vi "LVClass_HasoSlopes Set Slopes X.vi"(0 "HasoSlopes in":refnum<class "HasoSlopes.lvclass">, 5 "Slopesx":sgl[][](array[numeric]), 11 "error in (no error)":errorcluster) -> (4 "HasoSlopes out":refnum<class "HasoSlopes.lvclass">, 15 "error out":errorcluster)   [LabVIEW 2020, in "HasoSlopes.lvclass"]
doc: "HasoSlopes X coordinates getter.\n\n--------------------------------------------------------------------------------\n\n<B>HasoSlopesIn </B> : HasoSlopes object.\n<B>HasoSlopesOut </B> : HasoSlopes object.\n<B>slopes_x </B> : 2D slopes X buffer.\n<B>ErrorIn </B> : Error\n<B>ErrorOut </B> : Error\n\n--------------------------------------------------------------------------------"
uses:
  HasoSlopes.lvclass
  HasoSlopes.lvclass/HasoSlopes.ctl
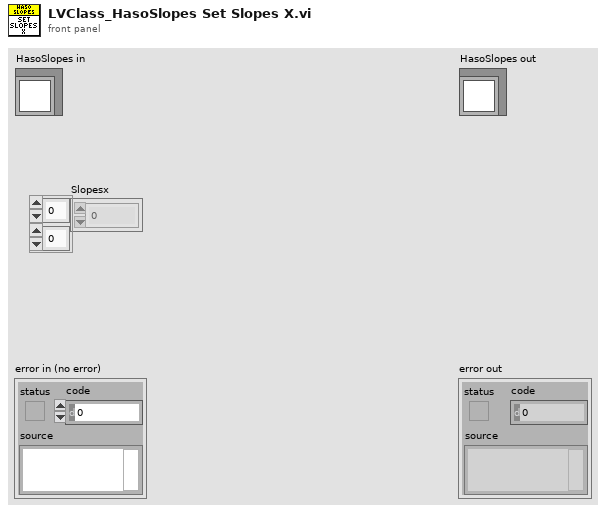
[diagram p1: front panel]
types:
  T1 = typedef "Point2D.ctl" = cluster{"X":u32, "Y":u32}
  T2 = typedef "Point2Df.ctl" = cluster{"X":sgl, "Y":sgl}
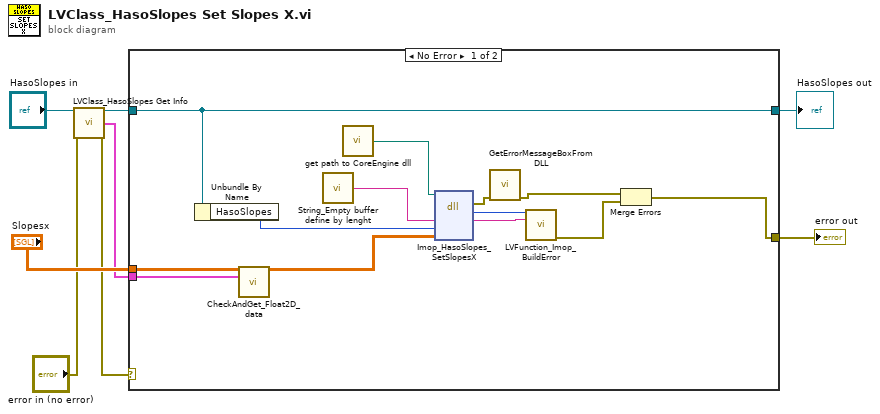
[diagram p0: block diagram]
diagram:
  n1 = call "LVClass_HasoSlopes Get Info.vi"("HasoSlopes in"="HasoSlopes in", "error in (no error)"="error in (no error)") -> ("HasoSlopes out"=w1:refnum<class "HasoSlopes.lvclass">, "dimension"=w5:cluster{"size":T1, "step":T2}, "error out"=w3:errorcluster)  [unwired: 9 in, 2 out]
  n2 = case shown="No Error" w3 {
    selector: w3 -> [_ w23]
    tunnel: [w12 w23] -> w8
    tunnel: [w15 w22] -> w7
    tunnel: w1 -> [w15 w22]
    tunnel: "Slopesx" -> [w11 _]
    tunnel: w5 -> [w9 _]
    frame No Error {
      n3 = Unbundle By Name(w15) -> ("HasoSlopes"=w18:i32)
      n4 = call "CheckAndGet_Float2D_data.vi"("data in"=w11, "Dimensions_um"=w9) -> ("data out"=w10:sgl[][])  [unwired: 13 in]
      n5 = call "String_Empty buffer define by lenght.vi"() -> ("Empty buffer"=w21:string)  [unwired: 1 in]
      n6 = call "get path to CoreEngine dll.vi"() -> ("path to c_interface_vc100.dll"=w17:path)  [unwired: 12 in, 3 out]
      n7 = dll-call lib="D:/2_trunk/Soft_haso/ImOpCoreEngine4_LV2011/DLLs/ImopEngine4_vc100.dll" fn="Imop_HasoSlopes_SetSlopesX"(path in=w17, "message"=w21, "objet"=w18, "Slopesx"=w10) -> (error out=w16:errorcluster, "return type"=w19:i32, "message"=w20:string)  [unwired: 4 in, 1 out]
      n8 = call "GetErrorMessageBoxFromDLL.vi"("error IN"=w16) -> ("error OUT"=w14:errorcluster)  [unwired: 10 in]
      n9 = call "LVFunction_Imop_BuildError.vi"("code"=w19, "String to Prepend to source (\"\")"=w20) -> ("error out"=w13:errorcluster)  [unwired: 13 in]
      n10 = Merge Errors(w14, w13) -> (w12:errorcluster)
    }
    frame Error {
    }
  }
  "error out" <- w8
  "HasoSlopes out" <- w7
